vi "Set-Background-correction.vi"(8 "error in (no error)":errorcluster, 10 "Correct. params in":refnum<data-value>, 11 "Camera in":refnum<class "Camera.lvclass">) -> (0 "error out":errorcluster, 2 "Correct. params":refnum<data-value>, 3 "Camera out":refnum<class "Camera.lvclass">)   [LabVIEW 2013, in "CameraVision.lvlib" / "Camera.lvclass"]
uses:
  Camera.lvclass
  Main/Correction/CV-Correction.lvclass
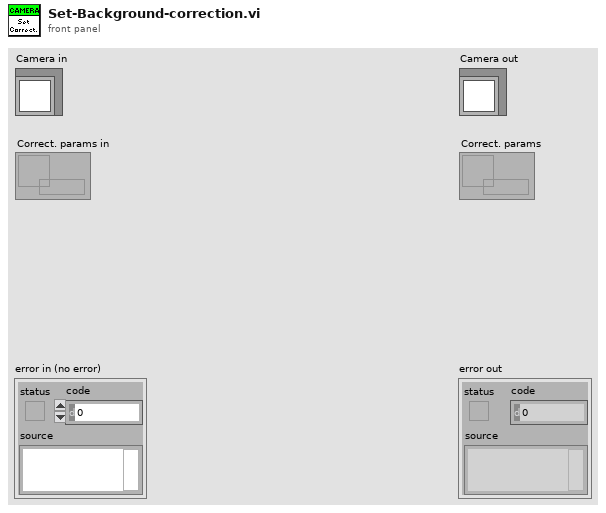
[diagram p1: front panel]
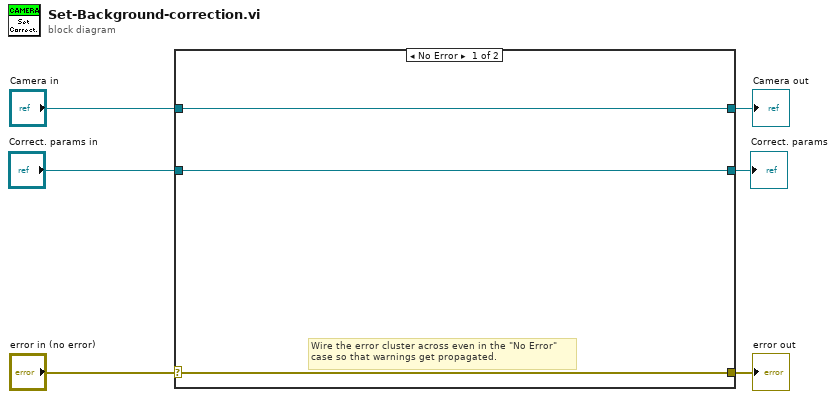
[diagram p0: block diagram]
diagram:
  n1 = case shown="No Error" "error in (no error)" {
    selector: "error in (no error)" -> [w8 w12]
    tunnel: [w8 w12] -> w5
    tunnel: [w9 w11] -> w3
    tunnel: "Camera in" -> [w9 w11]
    tunnel: "Correct. params in" -> [w7 w10]
    tunnel: [w7 w10] -> w1
    frame No Error {
      # "Wire the error cluster across even in the \"No Error\"\ncase so that warnings get propagated."
    }
    frame Error {
    }
  }
  "error out" <- w5
  "Camera out" <- w3
  "Correct. params" <- w1
